vi "ClockSyncPayload.vi"(5 "T1":i64, 9 "T2":i64) -> (8 "JSON string":string)   [LabVIEW 2020, in "epl-network.lvlib"]
uses:
  epl-network.lvlib
  ClockSyncPayload.ctl
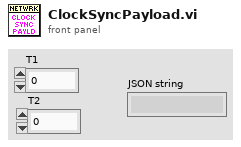
[diagram p1: front panel]
types:
  T1 = typedef "epl-network.lvlib/ClockSyncPayload.ctl" = cluster{"T1":i64, "T2":i64}
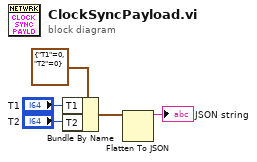
[diagram p0: block diagram]
diagram:
  n1 = Bundle By Name(cluster=T1 {"T1"=0, "T2"=0} ("ClockSyncPayload"), "T1"="T1", "T2"="T2") -> (w2:T1)
  n2 = Flatten To JSON(anything=w2) -> (JSON string=→"JSON string":string)  [unwired: 2 in, 1 out]
